vi "batch_processor_small.vi"() -> ()   [LabVIEW 2013]
uses:
  <vilib>/Utility/miscctls.llb/LVPointTypeDef.ctl
  Private/File_location.ctl
  Batch Processor/bp_cluster.ctl
  <vilib>/Utility/error.llb/DialogType.ctl
  Public API/Signal.ctl
  Private/Role ID.ctl
  Private/Hardware ID.ctl
  Public API/Post_Dust_Event.ctl
  Private/Estimate_source.ctl
panel:
  in  "Tab Control":enum32{"Controls", "Processing"}(tab)
  in  "Update old Errored entries?":bool
  in  "Clear IDL Errors 2":bool
  in  "Clear IDL Errors":bool
  out "Warning:":string
  out "Move Errors":errorcluster
  out "IDL Errors":errorcluster
  out "Test":bool caption="Test Database in use:"
  out "Test 2":bool=TRUE caption="Production Database in use:"
  out "Events being processed:":i32
  out "Processing Frequency (Hz):":dbl
  out "Database Update Progress:":u8(slide) scale=0.0..100.0
  out "IDL Code Executing":bool=TRUE
  out "Estimated IDL Progress:":u8(slide) scale=0.0..100.0
  in  "Update old database entries?":bool
  in  "Upper Timestamp\nFor Old Data":timestamp
  in  "Lower Timestamp\nFor Old Data":timestamp
  out "Running Old Data:":bool
  out "standard error":string
  out "standard output":string
  out "Quality":ext format="%.2f"
  out "Charge":ext
  out "Velocity":ext
  out "Source":i32
  out "Time taken by IDL per shot: (s)":dbl
  out "Shot being processed:":string
  out "Remaining Shots:":string
  out "Output to IDL command line:":string
  in  "stop":bool
  out "Radius":dbl
  out "Mass":ext
  out "Dust Event ID":i64
  # "Small Batch Processor"
  # "Error Status:"
  # "Beamline length change: 1:00:00.000 PM\n                                                       3/5/2014"
  # "ODBC Connection Status:"
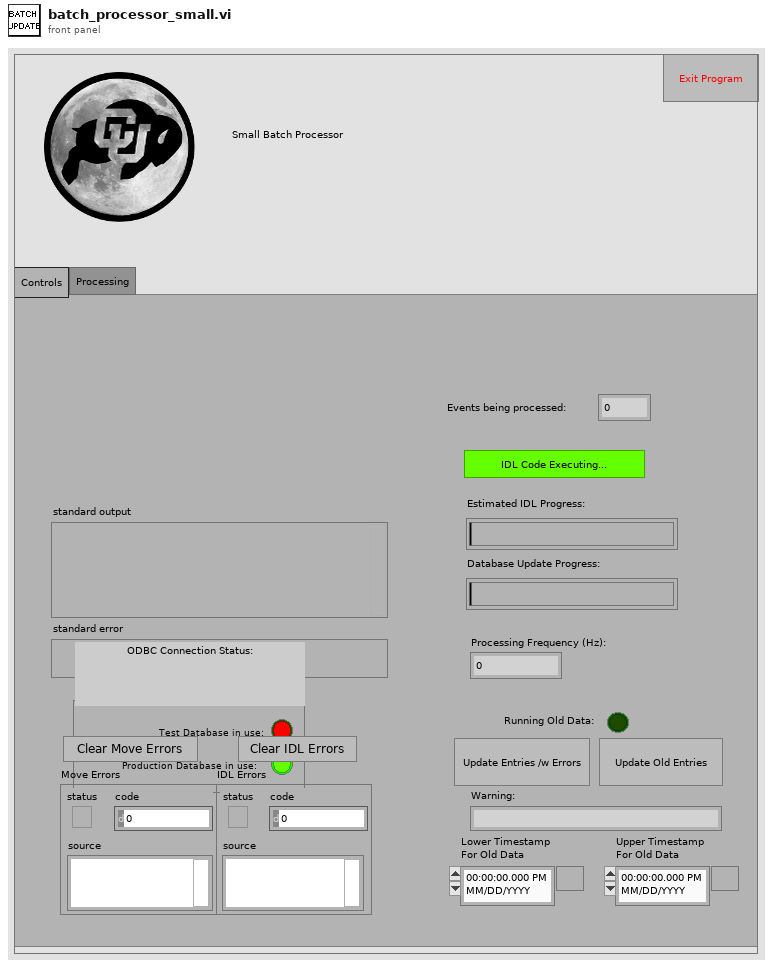
[diagram p1: front panel]
types:
  T1 = typedef "LVPointTypeDef.ctl" = cluster{"Horizontal":i16, "Vertical":i16}
  T2 = typedef "bp_cluster.ctl" = cluster{"Dust Event ID":i64, "High Voltage":sgl, "Experiment Settings  ID":i64, "File Location":T3, "Dust Density":dbl}
  T3 = typedef "File_location.ctl" = i8
  T4 = typedef "Signal.ctl" = cluster{"Signal ID":i64, "Time Stamp":timestamp, "Dust Event ID":i64, "Role ID":T5, "Data":sgl[], "Signal Length":i32, "dt":sgl, "Offset":dbl, "Hardware ID":T6}
  T5 = typedef "Role ID.ctl" = enum16{"First_Detector", "Second_Detector", "Third_Detector", "LeCroy_CH1", "LeCroy_CH2", "LeCroy_CH3", "LeCroy_CH4", "PSU"}
  T6 = typedef "Hardware ID.ctl" = enum16{"Unknown", "CSA 1", "CSA 2", "CSA 3", "CSA 4", "CSA 5", "CSA 6"}
  T7 = enum16{"open", "replace", "create", "open or create", "replace or create", "replace or create with confirmation"}
  T8 = typedef "Post_Dust_Event.ctl" = cluster{"Dust Event ID":i64, "Integer Timestamp":i64, "Velocity":sgl, "Mass":sgl, "Charge":sgl, "Radius":sgl, "Passed_3rd_Detector":i8, "Experiment Settings":dbl, "Pelletron ID":i32, "Estimate Source":T9, "Estimate Quality":sgl, "File Location":T3, "id_dust_info":dbl}
  T9 = typedef "Estimate_source.ctl" = i8
  T10 = enum8{"Enabled", "Disabled", "Disabled and Grayed Out"}
  T11 = typedef "DialogType.ctl" = u16
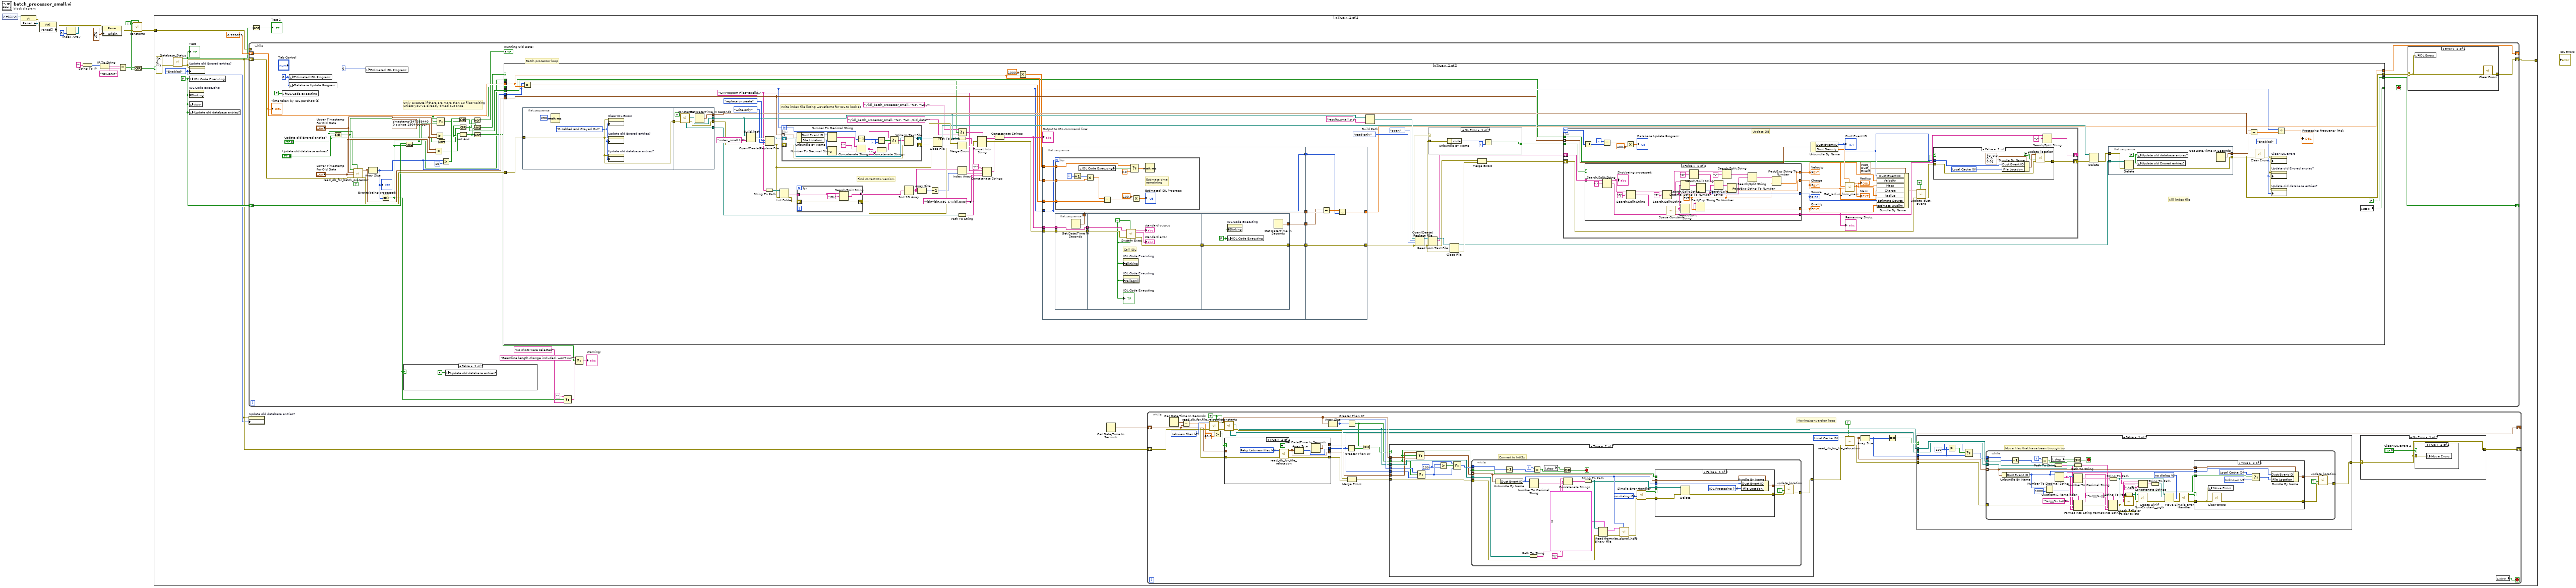
[diagram p0: block diagram]
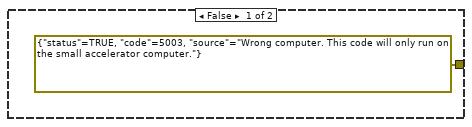
[diagram p2: hidden frame]
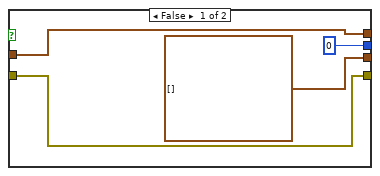
[diagram p3: hidden frame]
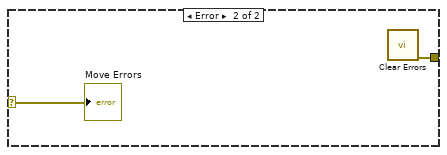
[diagram p5: hidden frame]
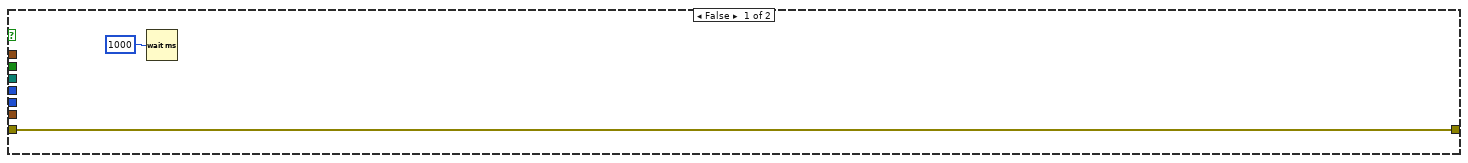
[diagram p6: hidden frame]
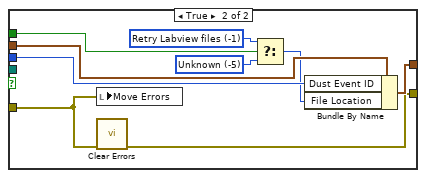
[diagram p7: hidden frame]
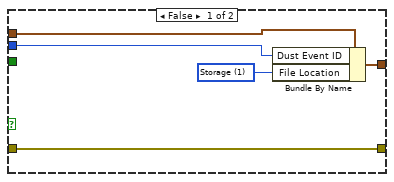
[diagram p8: hidden frame]
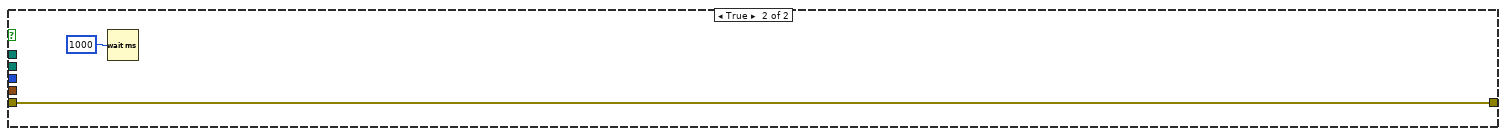
[diagram p9: hidden frame]
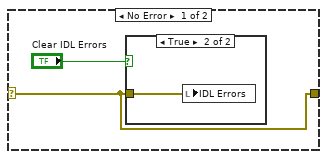
[diagram p10: hidden frame]
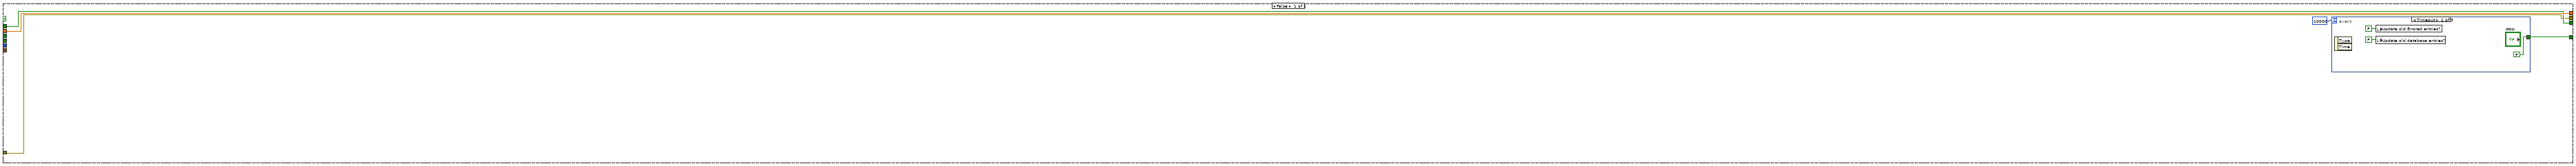
[diagram p13: hidden frame]
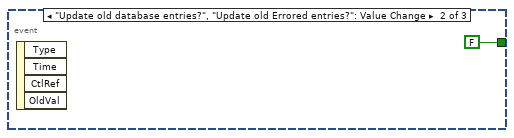
[diagram p14: hidden frame]
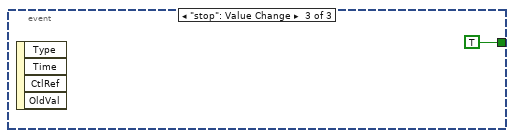
[diagram p15: hidden frame]
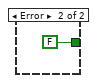
[diagram p16: hidden frame]
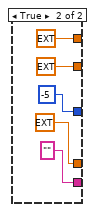
[diagram p18: hidden frame]
diagram:
  n1 = control-ref of="This VI"() -> (w18:refnum<vi>)
  n2 = property class="VI"(reference=w18) -> (error out=w17:errorcluster, "Panel"=w16:refnum<vi>)  [unwired: 1 in, 1 out]
  n3 = property class="Pnl"(reference=w16, error in=w17) -> (error out=w15:errorcluster, "Panes[]"=w14:refnum<vi>[])  [unwired: 1 out]
  n4 = Index Array(array=w14, index=0) -> (element=w12:refnum<vi>)
  n5 = String To IP(1:"" ("name")) -> (0:w10:u32)
  n6 = IP To String(2:w10) -> (0:w8:string)  [unwired: 1 in]
  n7 = property class="Pane"(reference=w12, error in=w15, "Origin"=T1 {"Horizontal"=0, "Vertical"=0}) -> (error out=w4:errorcluster)  [unwired: 1 out]
  n8 = Equal?(x=w8, y="NPL-PC-2") -> (x = y?=w6:bool)
  n9 = call "constants.vi"("error in (no error)"=w4, "Small?"=TRUE) -> ("error out"=w3:errorcluster, "Testing"=w2:bool)  [unwired: 3 in, 5 out]
  n10 = Or(x=w6, y=w2) -> (x .or. y?=w5:bool)
  n11 = case shown="True" w5 {
    tunnel: w3 -> [_ w25]
    tunnel: [errorcluster {"status"=TRUE, "code"=5003, "source"="Wrong computer. This code will only run on the small accelerator computer."} ("error IO") w20] -> _
    frame False {
    }
    frame True {
      w22 = T10."Enabled" ("Disabled")
      w29 = FALSE ("IDL Code Executing")
      n12 = call "Database_Status.vi"("error in (no error)"=errorcluster {"status"=FALSE, "code"=0, "source"=""}) -> ("error out"=w23:errorcluster, "Test Database"=w26:bool)  [unwired: 9 in]
      "Test" <- w26
      n13 = property on="Update old Errored entries?" class="Bool (strict)"(error in=w23, "DisabledEnum"=w22) -> ()  [unwired: 1 in, 2 out]
      n14 = local write "IDL Code Executing"(w29) -> ()
      n15 = property on="IDL Code Executing" class="Bool (strict)"("Blinking"=w29) -> ()  [unwired: 2 in, 2 out]
      n16 = local write "stop"(w29) -> ()
      n17 = local write "Update old database entries?"(w29) -> ()
      n18 = while {
        shift-right: [w233] -> _
        shift-left: sgl 0.53303 ("y") -> [w234]
        shift-right: [w228] -> _
        shift-left: w29 -> [w229]
        tunnel: w25 -> [_]
        shift-right: [w201] -> w20
        shift-left: w23 -> [w209]
        stop <- w231 stop-if-true
        w223 = timestamp(3476894400 s since 1904-01-01) ("y")
        w235 = u8 0 ("Database Update Progress")
        # "Only execute if there are more than 10 files waiting \nunless you've already timed out once"
        # "Batch processor loop"
        n19 = local write "IDL Code Executing"(FALSE ("IDL Code Executing")) -> ()
        n20 = local write "Estimated IDL Progress:"(w235) -> ()
        n21 = local write "Database Update Progress:"(w235) -> ()
        n22 = Or(x="Update old Errored entries?", y="Update old database entries?") -> (x .or. y?=w200:bool)
        n23 = call "read_db_for_batch_processor.vi"("Small?"=TRUE, "Update Error files?"="Update old Errored entries?", "error in (no error)"=w209, "Lower Timestamp"="Lower Timestamp\nFor Old Data", "Upper Timestamp"="Upper Timestamp\nFor Old Data", "Update old files?"=w200) -> ("error out"=w238:errorcluster, "BP Array"=w237:T2[])  [unwired: 4 in]
        n24 = local write "Estimated IDL Progress:"(u8 0 ("Estimated IDL Progress")) -> ()
        n25 = Array Size(array=w237) -> (size(s)=w226:i32)
        "Events being processed:" <- w226
        n26 = Not Equal To 0?(x=w226) -> (x != 0?=w205:bool)
        n27 = case shown="False" w205 {
          frame False {
            n28 = local write "Update old database entries?"(FALSE ("Update old database entries?")) -> ()
          }
          frame True {
          }
        }
        n29 = And(x=w229, y=w205) -> (x .and. y?=w206:bool)
        n30 = Greater?(x=w223, y="Lower Timestamp\nFor Old Data") -> (0:w220:bool)
        n31 = Greater?(x="Upper Timestamp\nFor Old Data", y=w223) -> (0:w219:bool)
        n32 = Select(t=w205, s=w200, f=w206) -> (s? t:f=w207:bool)
        n33 = Not(x="Update old database entries?") -> (.not. x?=w210:bool)
        n34 = Greater?(x=w226, y=10) -> (0:w227:bool)
        n35 = Or(x=w227, y=w207) -> (x .or. y?=w225:bool)
        n36 = Or(x=w219, y=w210) -> (x .or. y?=w211:bool)
        n37 = Not And(1:w219, 2:w220) -> (0:w218:bool)
        n38 = Not(x=w211) -> (.not. x?=→"Running Old Data:":bool)
        n39 = And(x=w225, y=w218) -> (x .and. y?=w221:bool)
        n40 = Not(x=w218) -> (.not. x?=w215:bool)
        n41 = case shown="True" w221 {
          tunnel: w238 -> [w245 w327]
          tunnel: [w245 w275] -> w202
          tunnel: w237 -> [_ w329]
          tunnel: w226 -> [_ w280]
          tunnel: w234 -> [w249 w292]
          tunnel: [w249 w288] -> w233
          tunnel: [w247 w285] -> w231
          tunnel: [w246 FALSE ("Update all files?")] -> w228
          tunnel: w205 -> [w246 _]
          tunnel: w211 -> [_ w276]
          tunnel: w200 -> [_ w255]
          frame False {
            n42 = event shown="[0] Timeout" {
              selector: _ -> [_ _ _]
              dyn-events: _ -> [_ _ _]
              timeout: u32 10000 ("milliseconds to wait") -> [_ _ _]
              tunnel: [FALSE FALSE TRUE] -> w247
              event Timeout {
                n43 = event-data() -> ()  [unwired: 1 in, 2 out]
                n44 = local write "Update old Errored entries?"(FALSE ("Update old Errored entries?")) -> ()
                n45 = local write "Update old database entries?"(FALSE ("Update old database entries?")) -> ()
              }
              event "Update old database entries?", "Update old Errored entries?": Value Change {
                n46 = event-data() -> ()  [unwired: 1 in, 4 out]
              }
              event "stop": Value Change {
                n47 = event-data() -> ()  [unwired: 1 in, 4 out]
              }
            }
          }
          frame True {
            w267 = "C:\\Program Files\\Exelis\\"
            w270 = T10."Enabled" ("Disabled")
            # "Find correct IDL version."
            # "Kill index file"
            # "Write index file listing waveforms for IDL to look at"
            n48 = flat-sequence {
              tunnel: w327 -> [w340]
              tunnel: [w340] -> w284
              tunnel: [w346] -> w323
              tunnel: [w345] -> w304
              tunnel: [w344] -> w296
              tunnel: w284 -> [w347]
              tunnel: [w343] -> w282
              frame #0 {
                w339 = T10."Disabled and Grayed Out" ("Disabled")
                n49 = Wait (ms)(milliseconds to wait=u32 250) -> ()  [unwired: 1 out]
                n50 = property on="Clear IDL Errors" class="Bool"(error in=w340, "DisabledEnum"=w339) -> ()  [unwired: 1 in, 2 out]
                n51 = property on="Update old Errored entries?" class="Bool (strict)"(error in=w340, "DisabledEnum"=w339) -> ()  [unwired: 1 in, 2 out]
                n52 = property on="Update old database entries?" class="Bool (strict)"(error in=w340, "DisabledEnum"=w339) -> ()  [unwired: 1 in, 2 out]
              }
              frame #1 {
                n53 = call "constants.vi"("error in (no error)"=w347, "Small?"=TRUE) -> ("error out"=w346:errorcluster, "file path for Signal .hdf5 files"=w345:path, "file path for Processed Signal .hdf5 files"=w343:path)  [unwired: 3 in, 4 out]
                n54 = Get Date/Time In Seconds() -> (seconds since 1Jan1904=w344:timestamp)
              }
            }
            n55 = Multiply(x=w280, y=w292) -> (x*y=w294:dbl)
            n56 = Build Path(base path=w304, name or relative path="index_small.txt") -> (appended path=w326:path)
            n57 = String To Path(string=w267) -> (path=w266:path)
            n58 = Open/Create/Replace File(file path (use dialog)=w326, error in=w323, operation (0:open)=T7."replace or create", access (0:read/write)=enum16{"read/write", "read-only", "write-only"}."write-only") -> (refnum out=w325:refnum<file>, error out=w265:errorcluster)  [unwired: 2 in, 1 out]
            n59 = List Folder(path=w266, error in=w265) -> (folder names=w262:string[], error out=w263:errorcluster)  [unwired: 2 in, 2 out]
            n60 = for {
              N: w280 -> [w404]
              shift-right: [w411] -> w322
              shift-left: w265 -> [w410]
              tunnel: w329 -> [w412] mode=indexing
              shift-right: [w408] -> w324
              shift-left: w325 -> [w409]
              i -> [w407]
              n61 = Unbundle By Name(w412) -> ("Dust Event ID"=w398:i64, "File Location"=w397:T3)
              n62 = Number To Decimal String(number=w398) -> (decimal integer string=w400:string)  [unwired: 1 in]
              n63 = Number To Decimal String(number=w397) -> (decimal integer string=w395:string)  [unwired: 1 in]
              n64 = Decrement(x=w404) -> (x-1=w403:i32)
              n65 = Concatenate Strings(w400, " " ("string"), w395) -> (w399:string)
              n66 = Equal?(x=w403, y=w407) -> (x = y?=w406:bool)
              n67 = Concatenate Strings(w399, "," ("string")) -> (w401:string)
              n68 = Select(t=w399, s=w406, f=w401) -> (s? t:f=w405:string)
              n69 = Write to Text File(file (use dialog)=w409, text=w405, error in=w410) -> (refnum out=w408:refnum<file>, error out=w411:errorcluster)  [unwired: 1 in, 1 out]
            }
            n70 = for {
              tunnel: w262 -> [w331] mode=indexing
              shift-right: [w333] -> w264
              shift-left: w263 -> [w333]
              tunnel: [w330] -> w260 mode=indexing
              n71 = Search/Split String(string=w331, search string/char (-)="IDL" ("Element Data")) -> (match + rest of string=w330:string)  [unwired: 1 in, 2 out]
            }
            n72 = Sort 1D Array(array=w260) -> (sorted array=w261:string[])
            n73 = Array Size(array=w261) -> (size(s)=w258:i32)
            n74 = Decrement(x=w258) -> (x-1=w257:i32)
            n75 = Close File(refnum=w324, error in=w265) -> (path=w302:path, error out=w321:errorcluster)
            n76 = Path To String(path=w304) -> (string=w305:string)
            n77 = Path To String(path=w282) -> (string=w281:string)
            n78 = Select(t="\"idl_batch_processor_small, '%s', '%s'\"" ("format string"), s=w276, f="\"idl_batch_processor_small, '%s', '%s', /old_data\"" ("format string")) -> (s? t:f=w278:string)
            n79 = Merge Errors(w322, w321, w264) -> (w311:errorcluster)
            n80 = Index Array(array=w261, index=w257) -> (element=w259:string)
            n81 = Format Into String(format string=w278, error in=w311, w305, w281) -> (resulting string=w320:string, error out=w312:errorcluster)  [unwired: 1 in]
            n82 = Concatenate Strings("\"" ("string"), w267, w259, "\\bin\\bin.x86_64\\idl.exe\" -e ") -> (w268:string)
            n83 = Concatenate Strings "Concatenate Strings"(w268, w320) -> (w319:string)
            "Output to IDL command line:" <- w319
            n84 = Multiply(x=sgl 1000.0 ("y"), y=w292) -> (x*y=w293:dbl)
            n85 = flat-sequence {
              tunnel: [w353] -> w290
              tunnel: [w359] -> w289
              tunnel: [w358] -> w287
              tunnel: [w357] -> w286
              tunnel: w280 -> [w359]
              tunnel: w293 -> [w360]
              tunnel: w292 -> [w361]
              tunnel: w294 -> [w362]
              tunnel: w312 -> [w363]
              tunnel: w319 -> [w364]
              tunnel: w290 -> [w394]
              tunnel: w289 -> [w392]
              tunnel: [w391] -> w288
              tunnel: w287 -> [w390]
              tunnel: [w390] -> w274
              tunnel: w286 -> [w389]
              frame #0 {
                n86 = for {
                  N: w359 -> [_]
                  tunnel: w362 -> [w372]
                  tunnel: w361 -> [w375]
                  tunnel: w360 -> [w366]
                  i -> [w376]
                  # "Estimate time \nremaining"
                  n87 = Increment(x=w376) -> (x+1=w374:i32)
                  n88 = local read "IDL Code Executing"() -> (w368:bool)
                  n89 = Multiply(x=w374, y=w375) -> (x*y=w373:dbl)
                  n90 = Divide(x=w373, y=w372) -> (x/y=w371:dbl)
                  n91 = Select(t=w366, s=w368, f=0.0) -> (s? t:f=w367:dbl)
                  n92 = Multiply(x=sgl 100.0, y=w371) -> (x*y=→"Estimated IDL Progress:":dbl)
                  n93 = Wait (ms)(milliseconds to wait=w367) -> ()  [unwired: 1 out]
                }
                n94 = flat-sequence {
                  tunnel: w363 -> [w378]
                  tunnel: w364 -> [w379]
                  tunnel: [w379] -> w355
                  tunnel: [w378] -> w354
                  tunnel: [w377] -> w353
                  tunnel: [w383] -> w356
                  tunnel: w355 -> [w385]
                  tunnel: w354 -> [w384]
                  tunnel: [w387] -> w357
                  tunnel: [w388] -> w358
                  tunnel: w356 -> [w388]
                  frame #0 {
                    n95 = Get Date/Time In Seconds() -> (seconds since 1Jan1904=w377:timestamp)
                  }
                  frame #1 {
                    w382 = TRUE ("wait until completion? (T)")
                    # "Call IDL"
                    n96 = property on="IDL Code Executing" class="Bool (strict)"("Blinking"=w382) -> ()  [unwired: 2 in, 2 out]
                    n97 = property on="IDL Code Executing" class="Bool (strict)"("Val(Sgnl)"=w382) -> ()  [unwired: 2 in, 2 out]
                    n98 = call <vilib>:"System Exec.vi"("run minimized? (F)"=w382, "wait until completion? (T)"=w382, "error in (no error)"=w384, "command line"=w385) -> ("error out"=w383:errorcluster, "standard error"=→"standard error":string, "standard output"=→"standard output":string)  [unwired: 4 in, 1 out]
                    "IDL Code Executing" <- w382
                  }
                  frame #2 {
                    w386 = FALSE ("IDL Code Executing")
                    n99 = property on="IDL Code Executing" class="Bool (strict)"("Blinking"=w386) -> ()  [unwired: 2 in, 2 out]
                    n100 = local write "IDL Code Executing"(w386) -> ()
                    n101 = Get Date/Time In Seconds() -> (seconds since 1Jan1904=w387:timestamp)
                  }
                }
              }
              frame #1 {
                n102 = Subtract(x=w389, y=w394) -> (x-y=w393:dbl)
                n103 = Divide(x=w393, y=w392) -> (x/y=w391:dbl)
              }
            }
            n104 = Build Path(base path=w304, name or relative path="results_small.txt") -> (appended path=w317:path)
            n105 = Open/Create/Replace File(file path (use dialog)=w317, error in=w274, operation (0:open)=T7."open", access (0:read/write)=enum16{"read/write", "read-only", "write-only"}."read-only") -> (refnum out=w316:refnum<file>, error out=w273:errorcluster)  [unwired: 2 in, 1 out]
            n106 = case shown="No Error" w274 {
              tunnel: w273 -> [w337 _]
              tunnel: [w334 FALSE] -> w272
              frame No Error {
                n107 = Unbundle By Name(w337) -> ("code"=w336:i32)
                n108 = Equal?(x=w336, y=7) -> (x = y?=w334:bool)
              }
              frame Error {
              }
            }
            n109 = Read from Text File(file (use dialog)=w316, error in=w273) -> (refnum out=w306:refnum<file>, text=w303:string, error out=w315:errorcluster)  [unwired: 2 in, 1 out]
            n110 = Close File(refnum=w306, error in=w273) -> (path=w301:path, error out=w314:errorcluster)
            n111 = Merge Errors(w315, w314) -> (w313:errorcluster)
            n112 = for {
              N -> [w426]
              shift-right: [w416] -> w299
              shift-left: w313 -> [w431]
              tunnel: w329 -> [w439] mode=indexing
              shift-right: [w423] -> _
              shift-left: w303 -> [w432]
              tunnel: w272 -> [w419]
              tunnel: w255 -> [w414]
              i -> [w430]
              # "Update DB"
              n113 = Decrement(x=w426) -> (x-1=w425:i32)
              n114 = case shown="False" w419 {
                tunnel: [w463 -5] -> w438
                tunnel: [w449 ext 0.0] -> w437
                tunnel: [w461 ext -5.0] -> w418
                tunnel: [w450 ext -5.0] -> w434
                tunnel: w432 -> [w460 _]
                tunnel: [w455 ""] -> w424
                frame False {
                  w462 = ext 0.0 ("default (0 I32)")
                  n115 = Search/Split String(string=w460, search string/char (-)=",") -> (substring before match=w448:string, match + rest of string=w455:string)  [unwired: 1 in, 1 out]
                  "Shot being processed:" <- w448
                  n116 = Search/Split String(string=w448, search string/char (-)="Q") -> (substring before match=w470:string, match + rest of string=w471:string)  [unwired: 1 in, 1 out]
                  n117 = Search/Split String(string=w470, search string/char (-)="S") -> (substring before match=w452:string, match + rest of string=w468:string)  [unwired: 1 in, 1 out]
                  n118 = call <vilib>:"Space Constant.vi"() -> ("String"=w451:string)
                  n119 = Search/Split String(string=w468, search string/char (-)=w451) -> (match + rest of string=w454:string)  [unwired: 1 in, 2 out]
                  n120 = Search/Split String(string=w471, search string/char (-)=w451) -> (match + rest of string=w453:string)  [unwired: 1 in, 2 out]
                  n121 = Search/Split String(string=w452, search string/char (-)="C") -> (substring before match=w467:string, match + rest of string=w464:string)  [unwired: 1 in, 1 out]
                  n122 = Fract/Exp String To Number(string=w453, default (0 dbl)=w462) -> (number=w449:ext)  [unwired: 2 in, 1 out]
                  n123 = Decimal String To Number(string=w454) -> (number=w463:i32)  [unwired: 2 in, 1 out]
                  n124 = Search/Split String(string=w464, search string/char (-)=w451) -> (match + rest of string=w458:string)  [unwired: 1 in, 2 out]
                  n125 = Search/Split String(string=w467, search string/char (-)="V") -> (match + rest of string=w465:string)  [unwired: 1 in, 2 out]
                  n126 = Fract/Exp String To Number(string=w458, default (0 dbl)=w462) -> (number=w450:ext)  [unwired: 2 in, 1 out]
                  n127 = Search/Split String(string=w465, search string/char (-)=w451) -> (match + rest of string=w457:string)  [unwired: 1 in, 2 out]
                  n128 = Fract/Exp String To Number(string=w457, default (0 dbl)=w462) -> (number=w461:ext)  [unwired: 2 in, 1 out]
                }
                frame True {
                }
              }
              "Quality" <- w437
              "Charge" <- w434
              "Velocity" <- w418
              "Remaining Shots:" <- w424
              "Source" <- w438
              n129 = Divide(x=w430, y=w425) -> (x/y=w429:dbl)
              n130 = Multiply(x=w429, y=100.0) -> (x*y=→"Database Update Progress:":dbl)
              n131 = Unbundle By Name(w439) -> ("Dust Event ID"=w415:i64, "Dust Density"=w420:dbl)
              "Dust Event ID" <- w415
              n132 = call "Get_radius_from_mass.vi"("Density"=w420, "Charge"=w434, "Velocity"=w418) -> ("Mass"=w433:ext, "Radius"=w436:dbl)  [unwired: 7 in]
              "Mass" <- w433
              "Radius" <- w436
              n133 = Bundle By Name(cluster=T8 {"Dust Event ID"=0, "Integer Timestamp"=0, "Velocity"=0.0, "Mass"=0.0, "Charge"=0.0, "Radius"=0.0, "Passed_3rd_Detector"=0, "Experiment Settings"=0.0, "Pelletron ID"=0, "Estimate Source"=0, "Estimate Quality"=0.0, "File Location"=0, "id_dust_info"=0.0} ("Cluster"), "Dust Event ID"=w415, "Velocity"=w418, "Mass"=w433, "Charge"=w434, "Radius"=w436, "Estimate Source"=w438, "Estimate Quality"=w437) -> (w421:T8)
              n134 = call "update_dust_event.vi"("Small?"=TRUE, "error in (no error)"=w431, "Cluster"=w421) -> ("error out"=w417:errorcluster)  [unwired: 7 in, 1 out]
              n135 = case shown="False" w414 {
                tunnel: w417 -> [w446 w447]
                tunnel: [w445 w447] -> w416
                tunnel: w415 -> [w442 _]
                frame False {
                  w443 = T3 0 items=["IDL Processing"=-3, "Labview Files"=-2, "Unknown"=-1, "Local Cache "=0, "Old Storage"=1, "Storage"=2] ("File Location")
                  n136 = Bundle By Name(cluster=T2 {"Dust Event ID"=0, "High Voltage"=0.0, "Experiment Settings  ID"=0, "File Location"=0, "Dust Density"=0.0} ("Batch Processing Cluster"), "Dust Event ID"=w442, "File Location"=w443) -> (w441:T2)
                  n137 = call "update_location.vi"("error in (no error)"=w446, "Small?"=TRUE, "Batch Processing Cluster"=w441) -> ("error out"=w445:errorcluster)  [unwired: 7 in, 1 out]
                }
                frame True {
                }
              }
              n138 = Search/Split String(string=w424, search string/char (-)="V") -> (match + rest of string=w423:string)  [unwired: 1 in, 2 out]
            }
            n139 = Delete(path (use dialog)=w302, error in=w299) -> (error out=w300:errorcluster)  [unwired: 3 in, 2 out]
            n140 = flat-sequence {
              tunnel: w301 -> [w352]
              tunnel: w300 -> [w351]
              tunnel: [w350] -> w275
              tunnel: [w349] -> w297
              frame #0 {
                w348 = FALSE ("Update all files?")
                n141 = Delete(path (use dialog)=w352, error in=w351) -> (error out=w350:errorcluster)  [unwired: 3 in, 2 out]
                n142 = local write "Update old database entries?"(w348) -> ()
                n143 = local write "Update old Errored entries?"(w348) -> ()
                n144 = Get Date/Time In Seconds() -> (seconds since 1Jan1904=w349:timestamp)
              }
            }
            n145 = Subtract(x=w297, y=w296) -> (x-y=w298:dbl)
            n146 = call <vilib>:"Clear Errors.vi"("error in (no error)"=w275) -> ("error out"=w271:errorcluster)  [unwired: 6 in]
            n147 = property on="Clear IDL Errors" class="Bool"(error in=w271, "DisabledEnum"=w270) -> ()  [unwired: 1 in, 2 out]
            n148 = property on="Update old Errored entries?" class="Bool (strict)"(error in=w271, "DisabledEnum"=w270) -> ()  [unwired: 1 in, 2 out]
            n149 = property on="Update old database entries?" class="Bool (strict)"(error in=w271, "DisabledEnum"=w270) -> ()  [unwired: 1 in, 2 out]
            n150 = Divide(x=w280, y=w298) -> (x/y=→"Processing Frequency (Hz):":dbl)
            n151 = local read "stop"() -> (w285:bool)
          }
        }
        n152 = Select(t="" ("Warning:"), s=w205, f="No shots were selected") -> (s? t:f=w214:string)
        n153 = Select(t="Beamline length change included, won't run" ("Warning:"), s=w215, f=w214) -> (s? t:f=→"Warning:":string)
        n154 = case shown="Error" w202 {
          selector: w202 -> [w240 w243]
          tunnel: [w240 w242] -> w201
          frame No Error {
            n155 = case shown="True" "Clear IDL Errors" {
              tunnel: w240 -> [_ w241]
              frame False {
              }
              frame True {
                n156 = local write "IDL Errors"(w241) -> ()
              }
            }
          }
          frame Error {
            n157 = local write "IDL Errors"(w243) -> ()
            n158 = call <vilib>:"Clear Errors.vi"("error in (no error)"=w243) -> ("error out"=w242:errorcluster)  [unwired: 6 in]
          }
        }
        "Time taken by IDL per shot: (s)" <- w234
      }
      n159 = property on="Update old database entries?" class="Bool (strict)"(error in=w23, "DisabledEnum"=w22) -> ()  [unwired: 1 in, 2 out]
      n160 = Not(x=w26) -> (.not. x?=→"Test 2":bool)
      n161 = Get Date/Time In Seconds() -> (seconds since 1Jan1904=w21:timestamp)
      n162 = while {
        shift-right: [w48] -> _
        shift-left: w23 -> [w45]
        shift-right: [w33] -> _
        shift-left: w21 -> [w32]
        stop <- w61 stop-if-true
        w30 = TRUE ("Small?")
        w46 = T3 0 items=["IDL Processing"=-3, "Labview Files"=-2, "Mars Data Processing Factility"=-1, "Local Cache "=0, "Old Storage"=1, "Storage"=2] ("File Location")
        w53 = T3 -2 items=["Labview Files"=-2, "Mars Data Processing Factility"=-1, "Local Cache "=0, "Old Storage"=1, "Storage"=2] ("File Location")
        # "Moving/conversion loop"
        n163 = Get Date/Time In Seconds() -> (seconds since 1Jan1904=w37:timestamp)
        n164 = Subtract(x=w37, y=w32) -> (x-y=w36:dbl)
        n165 = call "read_db_for_file_relocation.vi"("Small?"=w30, "error in (no error)"=w45, "File Location"=w53) -> ("error out"=w57:errorcluster, "BP Array"=w55:T2[])  [unwired: 7 in]
        n166 = Greater?(x=w36, y=60.0) -> (0:w34:bool)
        n167 = call "constants.vi"("error in (no error)"=w57, "Small?"=w30) -> ("error out"=w56:errorcluster, "file path for Signal .hdf5 files"=w51:path, "file path for Processed Signal .hdf5 files"=w50:path)  [unwired: 3 in, 4 out]
        n168 = case shown="True" w34 {
          tunnel: w45 -> [w65 w72]
          tunnel: [w65 w71] -> w43
          tunnel: [T2[] [] ("BP Array") w70] -> w40
          tunnel: [0 w69] -> w38
          tunnel: [w63 w67] -> w33
          tunnel: w32 -> [w63 _]
          frame False {
          }
          frame True {
            w68 = T3 -1 items=["Unknown"=-5, "IDL Processing"=-4, "Writing from Queue"=-3, "Labview Files"=-2, "Retry Labview files"=-1, "Local Cache "=0, "Old Storage"=1, "Storage"=2] ("File Location")
            n169 = call "read_db_for_file_relocation.vi"("Small?"=TRUE, "error in (no error)"=w72, "File Location"=w68) -> ("error out"=w71:errorcluster, "BP Array"=w70:T2[])  [unwired: 7 in]
            n170 = Array Size(array=w70) -> (size(s)=w69:i32)
            n171 = Get Date/Time In Seconds() -> (seconds since 1Jan1904=w67:timestamp)
          }
        }
        n172 = Array Size(array=w55) -> (size(s)=w54:i32)
        n173 = Greater Than 0?(x=w38) -> (x > 0?=w41:bool)
        n174 = Greater Than 0?(x=w54) -> (x > 0?=w39:bool)
        n175 = Merge Errors(w56, w43) -> (w44:errorcluster)
        n176 = Or(x=w39, y=w41) -> (x .or. y?=w42:bool)
        n177 = case shown="True" w42 {
          tunnel: w44 -> [w78 w92]
          tunnel: w51 -> [_ w91]
          tunnel: w55 -> [_ w86]
          tunnel: w54 -> [_ w82]
          tunnel: [w78 w90] -> w52
          tunnel: w40 -> [_ w85]
          tunnel: w39 -> [_ w81]
          tunnel: w38 -> [_ w83]
          frame False {
            n178 = Wait (ms)(milliseconds to wait=u32 1000) -> ()  [unwired: 1 out]
          }
          frame True {
            w87 = 100 ("y")
            # "Convert to hdf5s"
            n179 = Select(t=w86, s=w81, f=w85) -> (s? t:f=w84:T2[])
            n180 = Select(t=w82, s=w81, f=w83) -> (s? t:f=w80:i32)
            n181 = Greater?(x=w80, y=w87) -> (0:w89:bool)
            n182 = Select(t=w87, s=w89, f=w80) -> (s? t:f=w88:i32)
            n183 = while {
              tunnel: w84 -> [w118] mode=indexing
              tunnel: w91 -> [w99]
              tunnel: w88 -> [w110]
              tunnel: w92 -> [w96]
              tunnel: [w119] -> w90
              tunnel: w81 -> [w97]
              i -> [w111]
              stop <- w114 stop-if-true
              w107 = T11 0 items=["no dialog", "OK message", "continue or stop message", "OK message + warnings", "continue/stop + warnings"] ("type of dialog (OK msg:1)")
              n184 = Unbundle By Name(w118) -> ("Dust Event ID"=w101:i64)
              n185 = Decrement(x=w110) -> (x-1=w112:i32)
              n186 = Path To String(path=w99) -> (string=w115:string)
              n187 = Number To Decimal String(number=w101) -> (decimal integer string=w95:string)  [unwired: 1 in]
              n188 = Equal?(x=w111, y=w112) -> (x = y?=w109:bool)
              n189 = local read "stop"() -> (w113:bool)
              n190 = Or(x=w113, y=w109) -> (x .or. y?=w114:bool)
              n191 = Concatenate Strings(w115, "\\" ("string"), w95) -> (w116:string)
              n192 = String To Path(string=w116) -> (path=w100:path)
              n193 = Read from Binary File(5:T4[] [] ("Signal array"), 8:w96, 11:w100) -> (0:w104:errorcluster, 2:w102:T4[])  [unwired: 3 in, 2 out]
              n194 = call "write_signal_hdf5.vi"("Index"=w101, "error in"=w104, "Signal array"=w102) -> ("error out"=w103:errorcluster)  [unwired: 7 in, 1 out]
              n195 = call <vilib>:"Simple Error Handler.vi"("type of dialog (OK msg:1)"=w107, "error in (no error)"=w103) -> ("error?"=w108:bool, "error out"=w106:errorcluster)  [unwired: 3 in, 3 out]
              n196 = case shown="False" w108 {
                tunnel: w118 -> [w126 w135]
                tunnel: [w125 w133] -> w117
                tunnel: w101 -> [w124 w134]
                tunnel: [w123 w132] -> w105
                tunnel: w106 -> [w122 w131]
                tunnel: w100 -> [w121 _]
                tunnel: w97 -> [_ w128]
                frame False {
                  w120 = T3 -4 items=["Unknown"=-5, "IDL Processing"=-4, "Writing from Queue"=-3, "Labview Files"=-2, "Retry Labview files"=-1, "Local Cache "=0, "Old Storage"=1, "Storage"=2] ("File Location")
                  n197 = Delete(path (use dialog)=w121, error in=w122) -> (error out=w123:errorcluster)  [unwired: 3 in, 2 out]
                  n198 = Bundle By Name(cluster=w126, "Dust Event ID"=w124, "File Location"=w120) -> (w125:T2)
                }
                frame True {
                  w127 = T3 -5 items=["Unknown"=-5, "IDL Processing"=-4, "Writing from Queue"=-3, "Labview Files"=-2, "Retry Labview files"=-1, "Local Cache "=0, "Old Storage"=1, "Storage"=2] ("f")
                  w130 = T3 -1 items=["Unknown"=-5, "IDL Processing"=-4, "Writing from Queue"=-3, "Labview Files"=-2, "Retry Labview files"=-1, "Local Cache "=0, "Old Storage"=1, "Storage"=2] ("File Location")
                  n199 = local write "Move Errors"(w131) -> ()
                  n200 = call <vilib>:"Clear Errors.vi"("error in (no error)"=w131) -> ("error out"=w132:errorcluster)  [unwired: 6 in]
                  n201 = Select(t=w130, s=w128, f=w127) -> (s? t:f=w129:T3)
                  n202 = Bundle By Name(cluster=w135, "Dust Event ID"=w134, "File Location"=w129) -> (w133:T2)
                }
              }
              n203 = call "update_location.vi"("error in (no error)"=w105, "Small?"=TRUE, "Batch Processing Cluster"=w117) -> ("error out"=w119:errorcluster)  [unwired: 7 in, 1 out]
            }
          }
        }
        n204 = call "read_db_for_file_relocation.vi"("Small?"=TRUE, "error in (no error)"=w52, "File Location"=w46) -> ("error out"=w49:errorcluster, "BP Array"=w60:T2[])  [unwired: 7 in]
        n205 = Array Size(array=w60) -> (size(s)=w58:i32)
        n206 = Equal To 0?(x=w58) -> (x = 0?=w59:bool)
        n207 = case shown="False" w59 {
          tunnel: w49 -> [w144 w197]
          tunnel: w50 -> [w143 _]
          tunnel: w51 -> [w142 _]
          tunnel: w60 -> [w141 _]
          tunnel: w58 -> [w137 _]
          tunnel: [w140 w197] -> w47
          frame False {
            w136 = 100 ("y")
            # "Move files that have been through bp"
            n208 = Greater?(x=w137, y=w136) -> (0:w139:bool)
            n209 = Select(t=w136, s=w139, f=w137) -> (s? t:f=w138:i32)
            n210 = while {
              tunnel: w141 -> [w181] mode=indexing
              tunnel: w143 -> [w178]
              tunnel: w142 -> [w179]
              tunnel: w138 -> [w172]
              tunnel: w144 -> [w170]
              tunnel: [w182] -> w140
              i -> [w173]
              stop <- w176 stop-if-true
              w163 = T11 0 items=["no dialog", "OK message", "continue or stop message", "OK message + warnings", "continue/stop + warnings"] ("type of dialog (OK msg:1)")
              n211 = Unbundle By Name(w181) -> ("Dust Event ID"=w160:i64)
              n212 = Decrement(x=w172) -> (x-1=w174:i32)
              n213 = Equal?(x=w173, y=w174) -> (x = y?=w171:bool)
              n214 = Quotient & Remainder(x=w160, y=i64 1000) -> (floor(x/y)=w159:i64)  [unwired: 1 out]
              n215 = local read "stop"() -> (w175:bool)
              n216 = Path To String(path=w179) -> (string=w151:string)
              n217 = Number To Decimal String(number=w160) -> (decimal integer string=w147:string)  [unwired: 1 in]
              n218 = Or(x=w175, y=w171) -> (x .or. y?=w176:bool)
              n219 = Path To String(path=w178) -> (string=w168:string)
              n220 = Number To Decimal String(number=w159) -> (decimal integer string=w157:string)  [unwired: 1 in]
              n221 = Format Into String(format string="%s\\\\%s.hdf5", error in=w170, w151, w147) -> (resulting string=w150:string, error out=w167:errorcluster)  [unwired: 1 in]
              n222 = String To Path(string=w150) -> (path=w156:path)
              n223 = Format Into String(format string="%s\\\\%s\\\\", error in=w167, w168, w157) -> (resulting string=w148:string, error out=w152:errorcluster)  [unwired: 1 in]
              n224 = String To Path(string=w148) -> (path=w153:path)
              n225 = call <vilib>:"Check if File or Folder Exists.vi"("error in (no error)"=w152, "path"=w156) -> ("file or folder exists?"=w155:bool)  [unwired: 7 in, 2 out]
              n226 = call <userlib>:"Create Dir if Non-Existant__ogtk.vi"("error in (no error)"=w152, "Directory Path"=w153) -> ("error out"=w154:errorcluster)  [unwired: 7 in, 2 out]
              n227 = Concatenate Strings(w148, w147, ".hdf5" ("string")) -> (w149:string)
              n228 = String To Path(string=w149) -> (path=w169:path)
              n229 = Move(source path=w156, error in=w154, 10:w169) -> (error out=w165:errorcluster)  [unwired: 2 in, 2 out]
              n230 = call <vilib>:"Simple Error Handler.vi"("type of dialog (OK msg:1)"=w163, "error in (no error)"=w165) -> ("error?"=w164:bool, "error out"=w162:errorcluster)  [unwired: 3 in, 3 out]
              n231 = case shown="True" w164 {
                tunnel: w181 -> [w187 w196]
                tunnel: [w186 w194] -> w180
                tunnel: w160 -> [w185 w195]
                tunnel: [w184 w193] -> w161
                tunnel: w162 -> [w184 w192]
                tunnel: w155 -> [_ w188]
                frame False {
                  w183 = T3 1 items=["Unknown"=-5, "IDL Processing"=-4, "Writing from Queue"=-3, "Labview Files"=-2, "Retry Labview files"=-1, "Local Cache "=0, "Storage"=1] ("File Location")
                  n232 = Bundle By Name(cluster=w187, "Dust Event ID"=w185, "File Location"=w183) -> (w186:T2)
                }
                frame True {
                  w189 = T3 -5 items=["Unknown"=-5, "IDL Processing"=-4, "Writing from Queue"=-3, "Labview Files"=-2, "Retry Labview files"=-1, "Local Cache "=0, "Old Storage"=1, "Storage"=2] ("f")
                  w191 = T3 0 items=["Currently Writing"=-3, "Labview Files"=-2, "Unknown"=-1, "Local Cache "=0, "Old Storage"=1, "Storage"=2] ("File Location")
                  n233 = local write "Move Errors"(w192) -> ()
                  n234 = call <vilib>:"Clear Errors.vi"("error in (no error)"=w192) -> ("error out"=w193:errorcluster)  [unwired: 6 in]
                  n235 = Select(t=w191, s=w188, f=w189) -> (s? t:f=w190:T3)
                  n236 = Bundle By Name(cluster=w196, "Dust Event ID"=w195, "File Location"=w190) -> (w194:T2)
                }
              }
              n237 = call "update_location.vi"("error in (no error)"=w161, "Small?"=TRUE, "Batch Processing Cluster"=w180) -> ("error out"=w182:errorcluster)  [unwired: 7 in, 1 out]
            }
          }
          frame True {
            n238 = Wait (ms)(milliseconds to wait=u32 1000) -> ()  [unwired: 1 out]
          }
        }
        n239 = case shown="No Error" w47 {
          selector: w47 -> [w73 w76]
          tunnel: [w73 w77] -> w48
          frame No Error {
            n240 = case shown="True" "Clear IDL Errors 2" {
              tunnel: w73 -> [_ w75]
              frame False {
              }
              frame True {
                n241 = local write "Move Errors"(w75) -> ()
              }
            }
          }
          frame Error {
            n242 = call <vilib>:"Clear Errors.vi"() -> ("error out"=w77:errorcluster)  [unwired: 7 in]
            "Move Errors" <- w76
          }
        }
        n243 = local read "stop"() -> (w61:bool)
      }
    }
  }
